vi "Flatten.vi"(8 "error in (no error)":errorcluster, 11 "Pulse Gen Basic Scan in":refnum<class "Pulse Gen Basic Scan.lvclass">) -> (0 "error out":errorcluster, 3 "Pulse Gen Basic Scan out":refnum<class "Pulse Gen Basic Scan.lvclass">)   [LabVIEW 2009, in "Pulse Gen Basic Scan.lvclass"]
uses:
  Pulse Gen Basic Scan.lvclass
  Scanner/Scanner.lvclass
  Pulse Gen Basic Scan.lvclass/Pulse Gen Basic Scan.ctl
  Global/File Locations.vi
panel:
  out "concatenated string":string
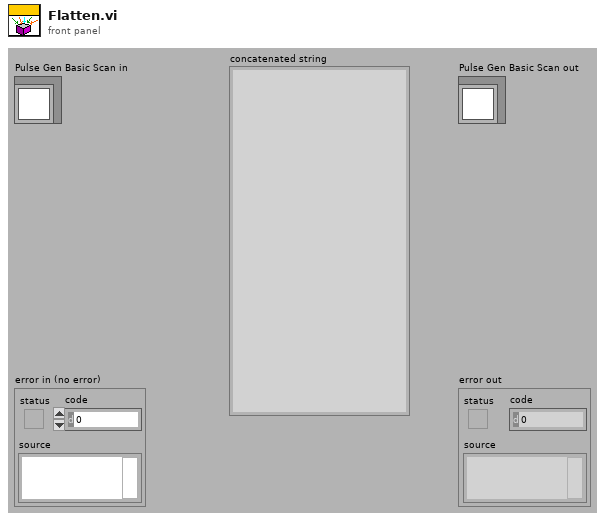
[diagram p1: front panel]
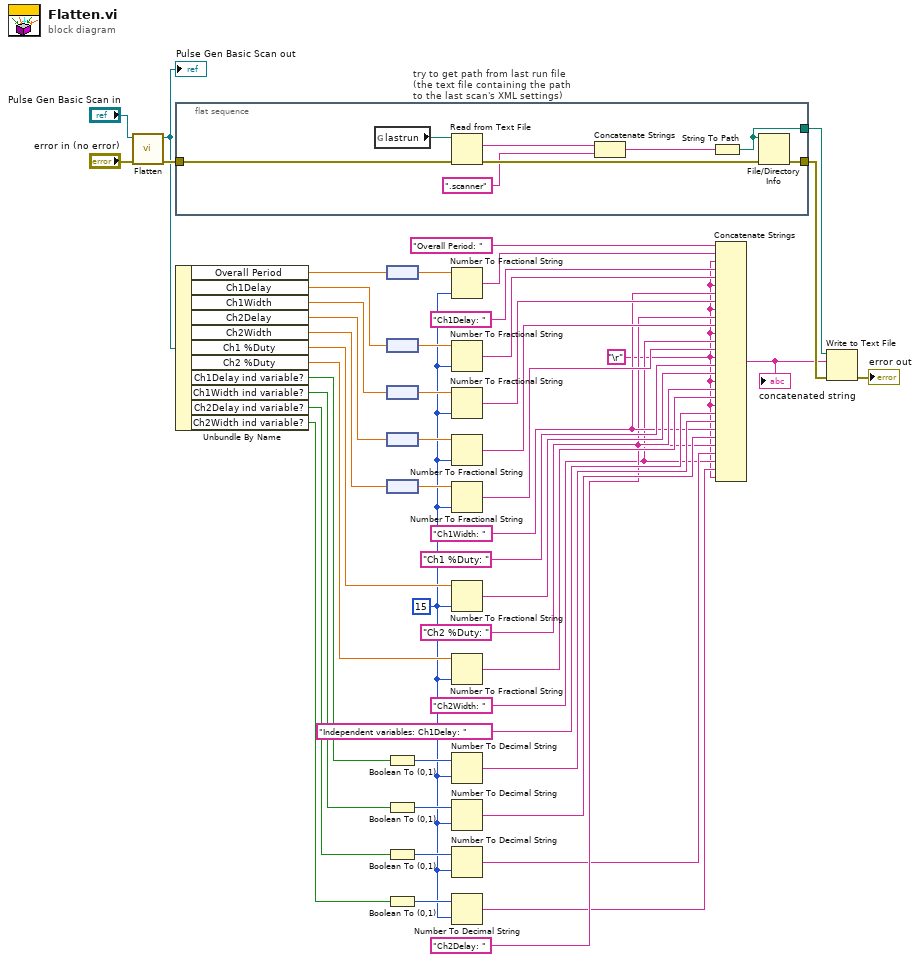
[diagram p0: block diagram]
diagram:
  w1 = 15
  w3 = "\r"
  w5 = "Ch2Width: "
  w7 = "Ch2Delay: "
  w8 = "Ch1Width: "
  n1 = call-parent "Flatten.vi"("error in (no error)"="error in (no error)", "Scanner in"="Pulse Gen Basic Scan in") -> ("error out"=w47:errorcluster, "Scanner out"=w43:refnum<class "Pulse Gen Basic Scan.lvclass">)  [unwired: 8 in]
  "Pulse Gen Basic Scan out" <- w43
  n2 = flat-sequence "try to get path from last run file\n(the text file containing the path\nto the last scan's XML settings)" {
    tunnel: [w57] -> w44
    tunnel: [w54] -> w45
    tunnel: w47 -> [w53]
    frame #0 {
      n3 = global read "File Locations.vi" "lastrun"() -> (w56:path)
      n4 = Read from Text File(file (use dialog)=w56, error in=w53) -> (text=w52:string, error out=w55:errorcluster)  [unwired: 4 out]
      n5 = Concatenate Strings(w52, ".scanner") -> (w50:string)
      n6 = String To Path(string=w50) -> (path=w57:path)
      n7 = File/Directory Info(path=w57, error in=w55) -> (error out=w54:errorcluster)  [unwired: 6 out]
    }
  }
  n8 = Unbundle By Name(w43) -> ("Overall Period"=w42:dbl[unit], "Ch1Delay"=w40:dbl[unit], "Ch1Width"=w37:dbl[unit], "Ch2Delay"=w36:dbl[unit], "Ch2Width"=w33:dbl[unit], "Ch1 %Duty"=w32:dbl, "Ch2 %Duty"=w31:dbl, "Ch1Delay ind variable?"=w19:bool, "Ch1Width ind variable?"=w18:bool, "Ch2Delay ind variable?"=w17:bool, "Ch2Width ind variable?"=w16:bool)
  n9 = node(w42) -> (w41:dbl)
  n10 = node(w40) -> (w39:dbl)
  n11 = node(w37) -> (w38:dbl)
  n12 = node(w36) -> (w35:dbl)
  n13 = node(w33) -> (w34:dbl)
  n14 = Boolean To (0,1)(Boolean=w19) -> (0, 1=w13:i16)
  n15 = Boolean To (0,1)(Boolean=w18) -> (0, 1=w12:i16)
  n16 = Boolean To (0,1)(Boolean=w17) -> (0, 1=w11:i16)
  n17 = Boolean To (0,1)(Boolean=w16) -> (0, 1=w10:i16)
  n18 = Number To Fractional String(number=w41, precision (6)=w1) -> (F-format string=w29:string)  [unwired: 2 in]
  n19 = Number To Fractional String(number=w39, precision (6)=w1) -> (F-format string=w27:string)  [unwired: 2 in]
  n20 = Number To Fractional String(number=w38, precision (6)=w1) -> (F-format string=w26:string)  [unwired: 2 in]
  n21 = Number To Fractional String(number=w35, precision (6)=w1) -> (F-format string=w25:string)  [unwired: 2 in]
  n22 = Number To Fractional String(number=w34, precision (6)=w1) -> (F-format string=w24:string)  [unwired: 2 in]
  n23 = Number To Fractional String(number=w32, precision (6)=w1) -> (F-format string=w22:string)  [unwired: 2 in]
  n24 = Number To Fractional String(number=w31, precision (6)=w1) -> (F-format string=w20:string)  [unwired: 2 in]
  n25 = Number To Decimal String(number=w13, width (-)=w1) -> (decimal integer string=w14:string)
  n26 = Number To Decimal String(number=w12, width (-)=w1) -> (decimal integer string=w9:string)
  n27 = Number To Decimal String(number=w11, width (-)=w1) -> (decimal integer string=w6:string)
  n28 = Number To Decimal String(number=w10, width (-)=w1) -> (decimal integer string=w4:string)
  n29 = Concatenate Strings("Overall Period: ", w29, w3, "Ch1Delay: ", w27, w3, w8, w26, w3, w7, w25, w3, w5, w24, w3, "Ch1 %Duty: ", w22, w3, "Ch2 %Duty: ", w20, w3, "Independent variables: Ch1Delay: ", w14, w8, w9, w7, w6, w5, w4, w3) -> (w2:string)
  "concatenated string" <- w2
  n30 = Write to Text File(file (use dialog)=w44, text=w2, error in=w45) -> (error out=→"error out":errorcluster)  [unwired: 1 in, 2 out]
